vi "Complete INT Task Order.vi"(8 "Error In":errorcluster) -> (0 "Error Out":errorcluster, 3 "Task Order":string)   [LabVIEW 2020, in "CollectionSupport.lvlib"]
uses:
  CollectionSupport.lvlib
panel:
  in  "OK Button":bool
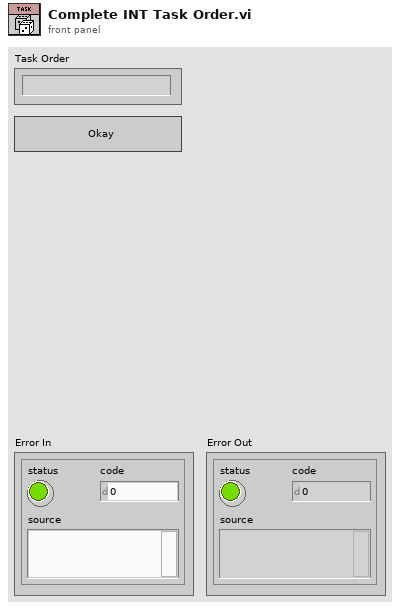
[diagram p1: front panel]
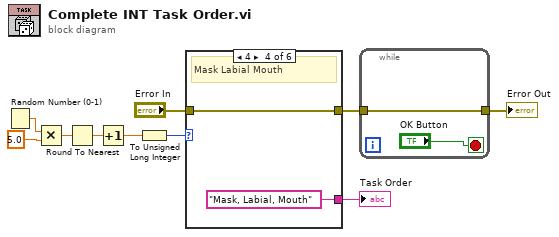
[diagram p0: block diagram]
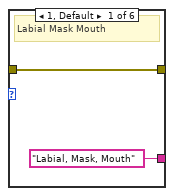
[diagram p2: hidden frame]
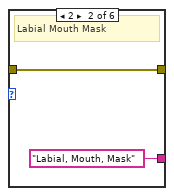
[diagram p3: hidden frame]
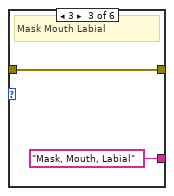
[diagram p4: hidden frame]
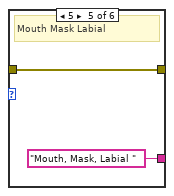
[diagram p5: hidden frame]
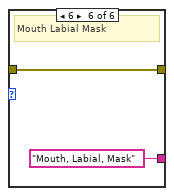
[diagram p6: hidden frame]
diagram:
  n1 = Random Number (0-1)() -> (number: 0 to 1=w10:dbl)
  n2 = Multiply(x=w10, y=5.0) -> (x*y=w8:dbl)
  n3 = Round To Nearest(number=w8) -> (nearest integer value=w7:dbl)
  n4 = Increment(x=w7) -> (x+1=w6:dbl)
  n5 = To Unsigned Long Integer(number=w6) -> (unsigned 32bit integer=w5:u32)
  n6 = case shown="4" w5 {
    tunnel: ["Labial, Mask, Mouth" "Labial, Mouth, Mask" "Mask, Mouth, Labial" "Mask, Labial, Mouth" "Mouth, Mask, Labial " "Mouth, Labial, Mask"] -> w4
    tunnel: "Error In" -> [w11 w13 w15 w17 w19 w21]
    tunnel: [w11 w13 w15 w17 w19 w21] -> w2
    frame 1, Default {
      # "Labial Mask Mouth"
    }
    frame 2 {
      # "Labial Mouth Mask"
    }
    frame 3 {
      # "Mask Mouth Labial"
    }
    frame 4 {
      # "Mask Labial Mouth"
    }
    frame 5 {
      # "Mouth Mask Labial"
    }
    frame 6 {
      # "Mouth Labial Mask"
    }
  }
  "Task Order" <- w4
  n7 = while {
    tunnel: w2 -> [w23]
    tunnel: [w23] -> w1
    stop <- "OK Button" stop-if-true
  }
  "Error Out" <- w1
